vi "RegisterCallback.vi"(8 "error in (no error)":errorcluster, 11 "service in":refnum<class "IcmMessageService.lvclass">) -> (0 "error out":errorcluster, 2 "callback":refnum<user-event>, 3 "service out":refnum<class "IcmMessageService.lvclass">)   [LabVIEW 2017, in "IcmMessageService.lvclass"]
doc: "Registers a callback to the message bus that causes the bus to return messages to the service. Wire the <B>callback</B> output this VI produces to the Register for Events function to register the callback as a source of events for an Event structure to monitor."
uses:
  <vilib>/addons/InsightCM/MessageBus/MessageService/IcmMessageService.lvclass
  <vilib>/addons/InsightCM/MessageBus/Base/controls/MessageWithState.ctl
  <vilib>/addons/InsightCM/MessageBus/Base/controls/Message.ctl
  <vilib>/addons/InsightCM/MessageBus/Base/controls/MessageHeader.ctl
  <vilib>/addons/InsightCM/MessageBus/Base/controls/KeyValuePair.ctl
  <vilib>/addons/InsightCM/MessageBus/MessageService/IcmMessageService.lvclass/IcmMessageService.ctl
  C:/Program Files (x86)/National Instruments/LabVIEW 2017/vi.lib/addons/InsightCM/Binaries/LabviewMessageAdapter.dll
  Binaries/LabviewMessageAdapter.dll
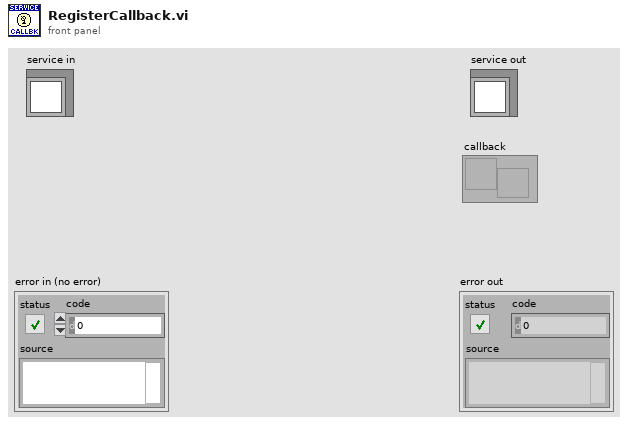
[diagram p1: front panel]
types:
  T1 = typedef "MessageWithState.ctl" = cluster{"Message":T2, "State":string}
  T2 = typedef "Message.ctl" = cluster{"Header":T3, "Body":u8[]}
  T3 = typedef "MessageHeader.ctl" = cluster{"MessageName":string, "Timestamp":i64, "CorrelationId":string, "ContentType":string, "RoutingKey":string, "Properties":T4[]}
  T4 = typedef "KeyValuePair.ctl" = cluster{"Key":string, "Value":string}
  T5 = typedef "MessageServiceDvr.ctl" = refnum<data-value>
  T6 = typedef "MessageServiceData.ctl" = cluster{"Service":refnum<k24>}
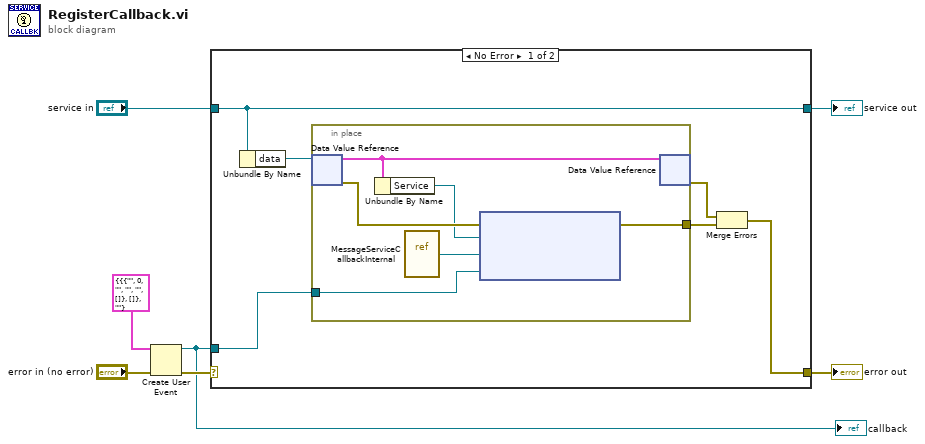
[diagram p0: block diagram]
diagram:
  n1 = Create User Event(user event datatype=T1 {"Message"={"Header"={"MessageName"="", "Timestamp"=0, "CorrelationId"="", "ContentType"="", "RoutingKey"="", "Properties"=[]}, "Body"=[]}, "State"=""} ("MessageWithState"), error in="error in (no error)") -> (user event=w1:refnum<user-event>, error out=w3:errorcluster)
  "callback" <- w1
  n2 = case shown="No Error" w3 {
    selector: w3 -> [_ w21]
    tunnel: [w9 w21] -> w7
    tunnel: [w13 w20] -> w5
    tunnel: "service in" -> [w13 w20]
    tunnel: w1 -> [w8 _]
    frame No Error {
      n3 = Unbundle By Name(w13) -> ("data"=w12:T5)
      n4 = in-place {
        in-place-border: [w17] -> w10
        in-place-border: w8 -> [w15]
        n5 = in-place-dvr #1(w12) -> (w19:T6, w18:errorcluster)
        n6 = Unbundle By Name(w19) -> ("Service"=w16:refnum<k24>)
        n7 = vi-ref <vilib>:"MessageServiceCallbackInternal.vi"() -> ("vi reference"=w14:refnum<vi>)
        n8 = node(w18, w16, w14, w15) -> (w17:errorcluster)  [unwired: 1 in, 1 out]
        n9 = in-place-dvr #1(w19) -> (w11:errorcluster)  [unwired: 1 out]
      }
      n10 = Merge Errors(w11, w10) -> (w9:errorcluster)
    }
    frame Error {
    }
  }
  "error out" <- w7
  "service out" <- w5
